vi "counterOrVolt.vi"(10 "element":u32 format="%032b") -> (1 "volt":bool, 2 "elementOut":u32 format="%032b")   [LabVIEW 2014]
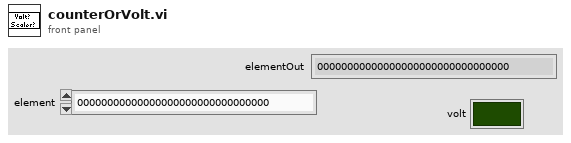
[diagram p1: front panel]
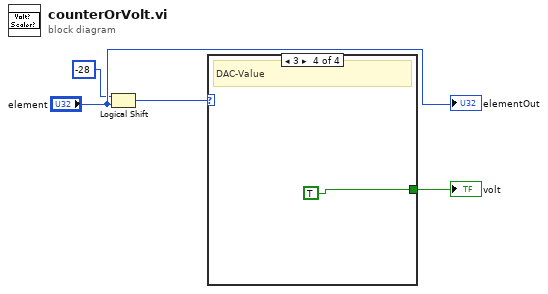
[diagram p0: block diagram]
diagram:
  n1 = Logical Shift(y=i16 -28, x="element") -> (x << y=w2:u32)
  n2 = case shown="3" w2 {
    tunnel: [_ _ _ TRUE ("volt")] -> w1
    frame 0, Default {
    }
    frame 1 {
      # "Simlcounter Value"
    }
    frame 2 {
      # "CS Seq Value"
    }
    frame 3 {
      # "DAC-Value"
    }
  }
  "volt" <- w1
  "elementOut" <- "element"
